vi "Teleop.vi"(10 "Match Info":T1={"Autonomous Elapsed Seconds"=0.0, "TeleOp Elapsed Seconds"=0.0, "Disabled Elapsed Seconds"=0.0, "Visited Autonomous"=FALSE, "Visited TeleOp"=FALSE, "Visited Disabled"=FALSE, "Autonomous Settings"={"Autonomous Style"=enum."Independent", "VI Refnum"=refnum}}, 11 "Call Context":T2) -> ()   [LabVIEW 2017]
doc: "This VI is called for each TeleOp packet received from the DS where the robot is not disabled. It is often used to read from the joysticks and update I/O or to update setpoints for timed control loops. It should complete and return within 20 milliseconds or it may miss DS packets."
uses:
  <vilib>/Rock Robotics/WPI/DriverStation/WPI_DriverStationDerivedRobotMode.ctl
  <vilib>/Rock Robotics/WPI/DriverStation/WPI_DriverStationMatch Info.ctl
  <vilib>/Rock Robotics/WPI/Utilities/WPI_GetSetVariantRefNum.vi
  <vilib>/Rock Robotics/Network Tables/NT Write Boolean Array.vi
  <vilib>/Rock Robotics/Network Tables/NT Write Numeric Array.vi
  <vilib>/Rock Robotics/Network Tables/NT Read Boolean.vi
  <vilib>/Rock Robotics/Network Tables/NT Read Number.vi
  Robot Global Data.vi
panel:
  out "Sample Slider 0":dbl(slide) scale=0.0..5.0
  out "Sample Boolean 1":bool
  out "Sample Boolean 0":bool
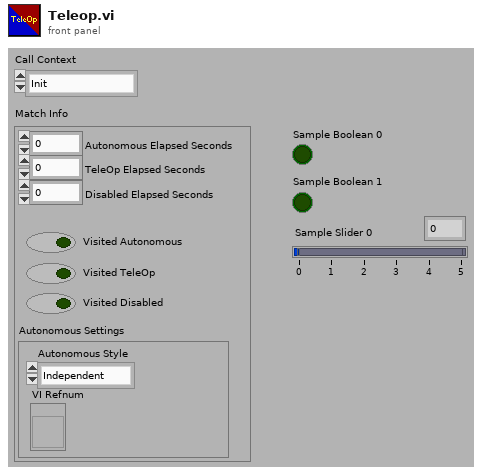
[diagram p1: front panel]
types:
  T1 = typedef "WPI_DriverStationMatch Info.ctl" = cluster{"Autonomous Elapsed Seconds":dbl, "TeleOp Elapsed Seconds":dbl, "Disabled Elapsed Seconds":dbl, "Visited Autonomous":bool, "Visited TeleOp":bool, "Visited Disabled":bool, "Autonomous Settings":cluster{"Autonomous Style":enum16{"Iterative", "Independent"}, "VI Refnum":refnum<vi>}}
  T2 = typedef "WPI_DriverStationDerivedRobotMode.ctl" = enum16{"Init", "Execute", "Stop"}
  T3 = typedef "WPI_MotorControlDeviceRef.ctl" = cluster{"DeviceStatus":errorcluster, "Type":T4, "PWM":cluster{"PWM Channel":T5, "DeadBand":T6}, "CAN":cluster{"Device Number":u8, "SetOutput VI Ref":variant, "GetOutput VI Ref":variant, "Enable VI Ref":variant, "Disable VI Ref":variant, "Data":variant}, "Invert":bool, "DIO PWM":cluster{"PWM \"Enable\" Channel":T5, "DIOChannel":T7, "PWM Rate":dbl}}
  T4 = typedef "WPI_MotorControlType.ctl" = enum16{"PWM", "CAN", "DIO PWM"}
  T5 = typedef "FPGA_DIOPWMChannel.ctl" = enum8{"PWM 0", "PWM 1", "PWM 2", "PWM 3", "PWM 4", "PWM 5", "PWM 6", "PWM 7", "PWM 8", "PWM 9", "PWM MXP 0", "PWM MXP 1", "PWM MXP 2", "PWM MXP 3", "PWM MXP 4", "PWM MXP 5", "PWM MXP 6", "PWM MXP 7", "PWM MXP 8", "PWM MXP 9", "Invalid"}
  T6 = typedef "WPI_PWMDeadband.ctl" = cluster{"Name":string, "maxPositivePwm":i32, "minPositivePwm":i32, "centerPwm":i32, "maxNegativePwm":i32, "minNegativePwm":i32, "angularRange":u16}
  T7 = typedef "FPGA_DIOChannel.ctl" = enum8{"DIO 0", "DIO 1", "DIO 2", "DIO 3", "DIO 4", "DIO 5", "DIO 6", "DIO 7", "DIO 8", "DIO 9", "DIO MXP 0", "DIO MXP 1", "DIO MXP 2", "DIO MXP 3", "DIO MXP 4", "DIO MXP 5", "DIO MXP 6", "DIO MXP 7", "DIO MXP 8", "DIO MXP 9", "DIO MXP 10", "DIO MXP 11", "DIO MXP 12", "DIO MXP 13", "DIO MXP 14", "DIO MXP 15", "SPI Port CS1", "SPI Port CS2", "SPI Port CS3", "SPI Port MISO", "SPI Port MOSI", "Invalid"}
  T8 = typedef "WPI_RobotDriveDevRef.ctl" = cluster{"DevStatus":errorcluster, "Motors[]":T3[], "Square Inputs":bool, "Max Output":dbl}
  T9 = typedef "WPI_JoystickDevRef.ctl" = cluster{"Device":T10}
  T10 = typedef "WPI_JoystickDeviceEnum.ctl" = enum16{"USB 0", "USB 1", "USB 2", "USB 3", "USB 4", "USB 5"}
  T11 = typedef "WPI_CompressorDevRef.ctl" = cluster{"DevStatus":errorcluster, "Pneumatics Control Module":u8}
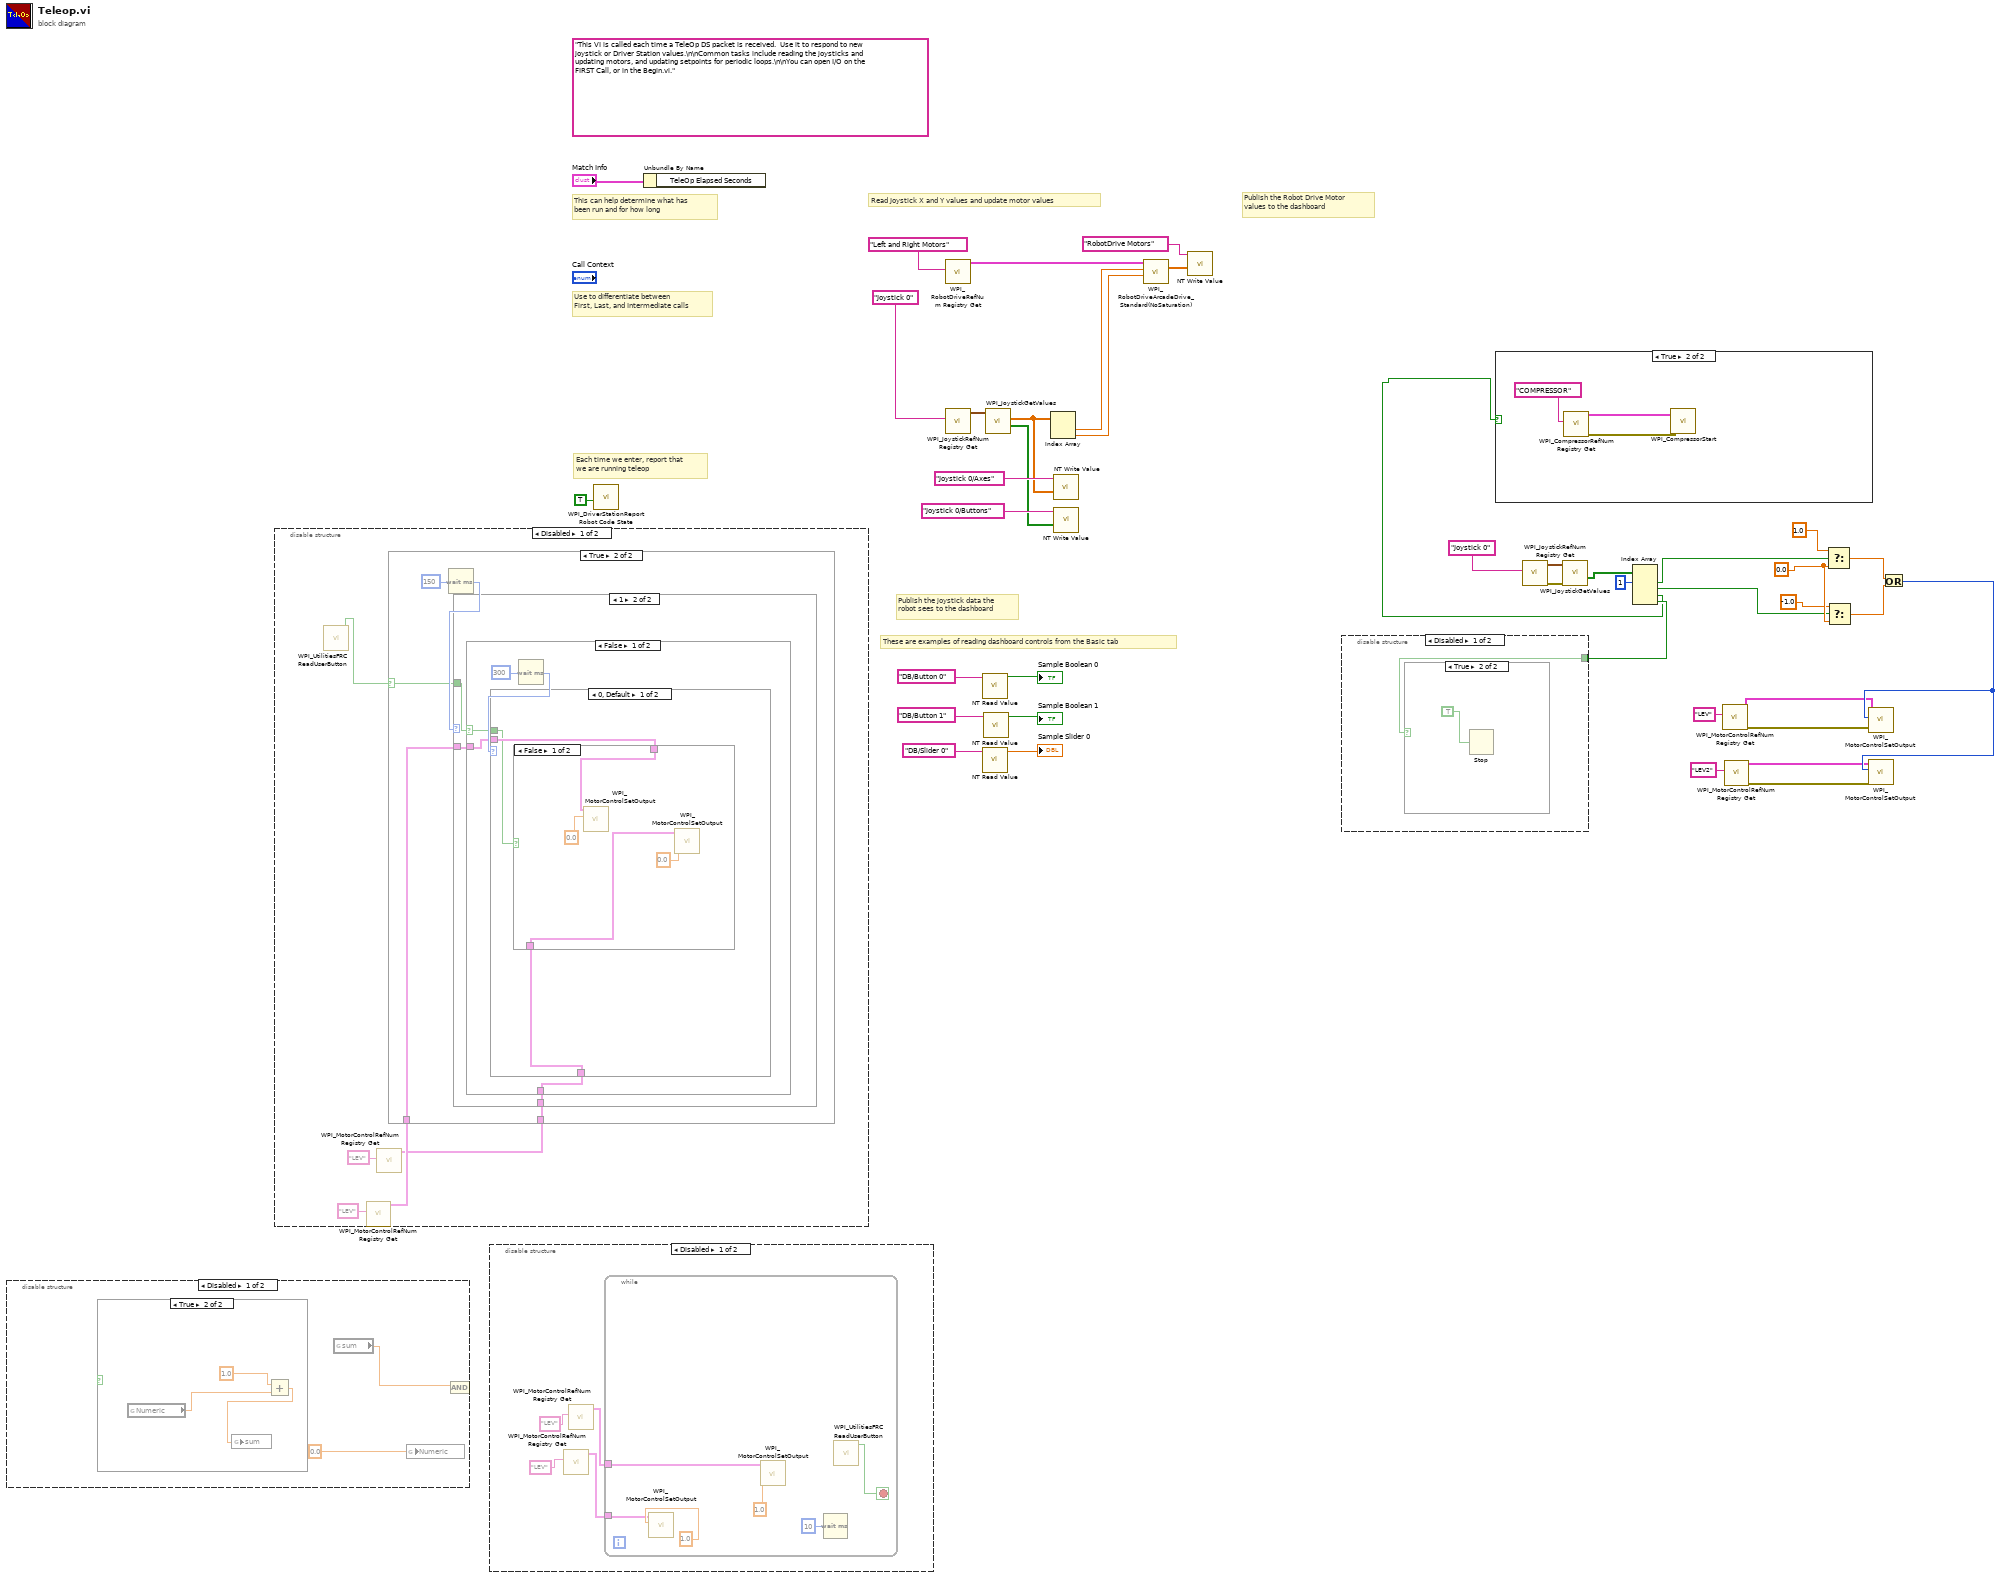
[diagram p0: block diagram]
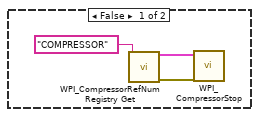
[diagram p4: hidden frame]
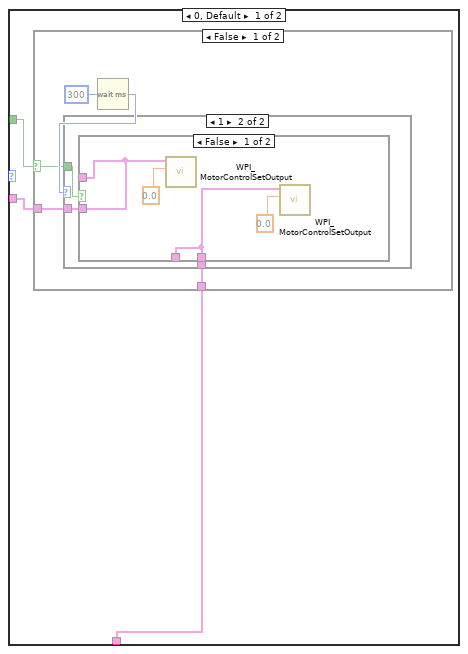
[diagram p9: hidden frame]
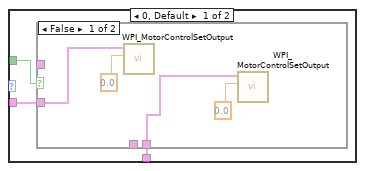
[diagram p10: hidden frame]
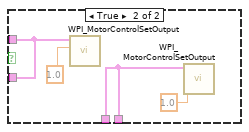
[diagram p11: hidden frame]
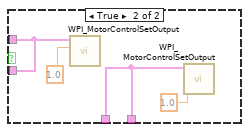
[diagram p12: hidden frame]
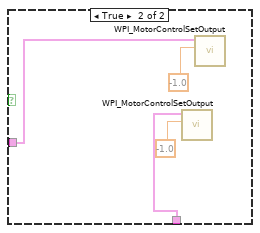
[diagram p13: hidden frame]
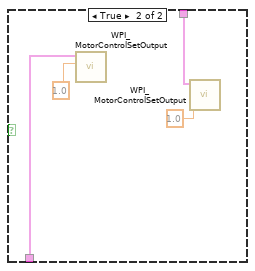
[diagram p14: hidden frame]
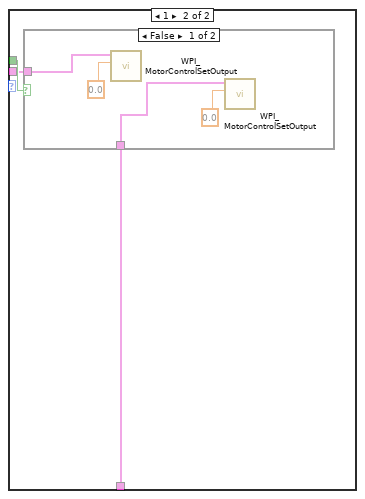
[diagram p15: hidden frame]
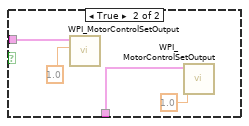
[diagram p16: hidden frame]
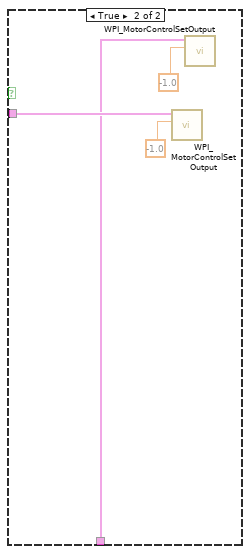
[diagram p17: hidden frame]
diagram:
  w16 = 0.0 ("t")
  (unwired) "This VI is called each time a TeleOp DS packet is received.  Use it to respond to new joystick or Driver Station values.\n\nCommon tasks include reading the joysticks and updating motors, and updating setpoints for periodic loops.\n\nYou can open I/O on the FIRST Call, or in the Begin.vi."
  # "Publish the Robot Drive Motor\nvalues to the dashboard"
  # "These are examples of reading dashboard controls from the Basic tab"
  # "Publish the joystick data the\nrobot sees to the dashboard"
  # "Each time we enter, report that\nwe are running teleop"
  # "Use to differentiate between\nFirst, Last, and Intermediate calls"
  # "This can help determine what has\nbeen run and for how long"
  # "Read Joystick X and Y values and update motor values"
  n1 = disable-structure shown="Disabled" {
    frame Disabled {
      n2 = case shown="True" {
        selector: _ -> [_ _]
        frame False {
        }
        frame True {
          n3 = global read "Robot Global Data.vi" "Numeric"() -> (w46:dbl)
          n4 = Add(x=1.0 ("Numeric"), y=w46) -> (x+y=w44:dbl)
          n5 = global write "Robot Global Data.vi" "sum"(w44) -> ()
        }
      }
      n6 = global read "Robot Global Data.vi" "sum"() -> (w42:dbl)
      n7 = global write "Robot Global Data.vi" "Numeric"(0.0 ("Numeric")) -> ()
      n8 = And(x=w42) -> ()  [unwired: 1 in, 1 out]
    }
    frame Enabled {
    }
  }
  n9 = disable-structure shown="Disabled" {
    frame Disabled {
      n10 = call <vilib>:"WPI_UtilitiesFRC ReadUserButton.vi"() -> ("User Button"=w51:bool)  [unwired: 10 in, 1 out]
      n11 = call <vilib>:"WPI_MotorControlRefNum Registry Get.vi"("refnum name"="LEV") -> ("MotorControlDevRef"=w48:T3)  [unwired: 9 in, 1 out]
      n12 = call <vilib>:"WPI_MotorControlRefNum Registry Get.vi"("refnum name"="LEV") -> ("MotorControlDevRef"=w47:T3)  [unwired: 9 in, 1 out]
      n13 = case shown="True" w51 {
        selector: w51 -> [_ w54]
        tunnel: w48 -> [_ w53]
        tunnel: w47 -> [_ w52]
        frame False {
        }
        frame True {
          n14 = Wait (ms)(milliseconds to wait=u32 150) -> (millisecond timer value=w56:u32)
          n15 = case shown="1" w56 {
            tunnel: w54 -> [w57 w93]
            tunnel: w53 -> [w59 w92]
            tunnel: w52 -> [w58 w91]
            frame 0, Default {
              n16 = case shown="False" w57 {
                selector: w57 -> [w62 _]
                tunnel: w59 -> [w61 w88]
                tunnel: w58 -> [w60 w87]
                frame False {
                  n17 = Wait (ms)(milliseconds to wait=u32 300) -> (millisecond timer value=w63:u32)
                  n18 = case shown="1" w63 {
                    tunnel: w62 -> [w67 w78]
                    tunnel: w61 -> [w66 w77]
                    tunnel: w60 -> [w65 w76]
                    frame 0, Default {
                      n19 = case shown="False" w67 {
                        tunnel: [_ w73] -> _
                        tunnel: [_ w72] -> _
                        tunnel: w66 -> [w69 w73]
                        tunnel: w65 -> [w68 w72]
                        frame False {
                          n20 = call <vilib>:"WPI_MotorControlSetOutput.vi"("Output"=0.0, "MotorControlDevRef"=w69) -> ()  [unwired: 7 in, 3 out]
                          n21 = call <vilib>:"WPI_MotorControlSetOutput.vi"("Output"=0.0, "MotorControlDevRef"=w68) -> ()  [unwired: 7 in, 3 out]
                        }
                        frame True {
                          n22 = call <vilib>:"WPI_MotorControlSetOutput.vi"("Output"=1.0, "MotorControlDevRef"=w73) -> ()  [unwired: 7 in, 3 out]
                          n23 = call <vilib>:"WPI_MotorControlSetOutput.vi"("Output"=1.0, "MotorControlDevRef"=w72) -> ()  [unwired: 7 in, 3 out]
                        }
                      }
                    }
                    frame 1 {
                      n24 = case shown="False" w78 {
                        tunnel: [w80 w83] -> _
                        tunnel: [w79 w84] -> _
                        tunnel: w77 -> [w80 w83]
                        tunnel: w76 -> [w79 w84]
                        frame False {
                          n25 = call <vilib>:"WPI_MotorControlSetOutput.vi"("Output"=0.0, "MotorControlDevRef"=w80) -> ()  [unwired: 7 in, 3 out]
                          n26 = call <vilib>:"WPI_MotorControlSetOutput.vi"("Output"=0.0, "MotorControlDevRef"=w79) -> ()  [unwired: 7 in, 3 out]
                        }
                        frame True {
                          n27 = call <vilib>:"WPI_MotorControlSetOutput.vi"("Output"=1.0, "MotorControlDevRef"=w83) -> ()  [unwired: 7 in, 3 out]
                          n28 = call <vilib>:"WPI_MotorControlSetOutput.vi"("Output"=1.0, "MotorControlDevRef"=w84) -> ()  [unwired: 7 in, 3 out]
                        }
                      }
                    }
                  }
                }
                frame True {
                  n29 = call <vilib>:"WPI_MotorControlSetOutput.vi"("Output"=-1.0, "MotorControlDevRef"=w87) -> ()  [unwired: 7 in, 3 out]
                  n30 = call <vilib>:"WPI_MotorControlSetOutput.vi"("Output"=-1.0, "MotorControlDevRef"=w88) -> ()  [unwired: 7 in, 3 out]
                }
              }
            }
            frame 1 {
              n31 = case shown="False" w93 {
                selector: w93 -> [w96 _]
                tunnel: w92 -> [w95 w123]
                tunnel: w91 -> [w94 w121]
                frame False {
                  n32 = Wait (ms)(milliseconds to wait=u32 300) -> (millisecond timer value=w97:u32)
                  n33 = case shown="0, Default" w97 {
                    tunnel: w96 -> [w99 w112]
                    tunnel: w95 -> [w100 w111]
                    tunnel: w94 -> [w101 w110]
                    frame 0, Default {
                      n34 = case shown="False" w99 {
                        tunnel: w101 -> [w103 w107]
                        tunnel: w100 -> [w102 w106]
                        frame False {
                          n35 = call <vilib>:"WPI_MotorControlSetOutput.vi"("Output"=0.0, "MotorControlDevRef"=w102) -> ()  [unwired: 7 in, 3 out]
                          n36 = call <vilib>:"WPI_MotorControlSetOutput.vi"("Output"=0.0, "MotorControlDevRef"=w103) -> ()  [unwired: 7 in, 3 out]
                        }
                        frame True {
                          n37 = call <vilib>:"WPI_MotorControlSetOutput.vi"("Output"=1.0, "MotorControlDevRef"=w107) -> ()  [unwired: 7 in, 3 out]
                          n38 = call <vilib>:"WPI_MotorControlSetOutput.vi"("Output"=1.0, "MotorControlDevRef"=w106) -> ()  [unwired: 7 in, 3 out]
                        }
                      }
                    }
                    frame 1 {
                      n39 = case shown="False" w112 {
                        tunnel: w111 -> [w113 w118]
                        tunnel: w110 -> [w114 w117]
                        frame False {
                          n40 = call <vilib>:"WPI_MotorControlSetOutput.vi"("Output"=0.0, "MotorControlDevRef"=w113) -> ()  [unwired: 7 in, 3 out]
                          n41 = call <vilib>:"WPI_MotorControlSetOutput.vi"("Output"=0.0, "MotorControlDevRef"=w114) -> ()  [unwired: 7 in, 3 out]
                        }
                        frame True {
                          n42 = call <vilib>:"WPI_MotorControlSetOutput.vi"("Output"=1.0, "MotorControlDevRef"=w118) -> ()  [unwired: 7 in, 3 out]
                          n43 = call <vilib>:"WPI_MotorControlSetOutput.vi"("Output"=1.0, "MotorControlDevRef"=w117) -> ()  [unwired: 7 in, 3 out]
                        }
                      }
                    }
                  }
                }
                frame True {
                  n44 = call <vilib>:"WPI_MotorControlSetOutput.vi"("Output"=-1.0, "MotorControlDevRef"=w123) -> ()  [unwired: 7 in, 3 out]
                  n45 = call <vilib>:"WPI_MotorControlSetOutput.vi"("Output"=-1.0, "MotorControlDevRef"=w121) -> ()  [unwired: 7 in, 3 out]
                }
              }
            }
          }
        }
      }
    }
    frame Enabled {
    }
  }
  n46 = disable-structure shown="Disabled" {
    frame Disabled {
      n47 = call <vilib>:"WPI_MotorControlRefNum Registry Get.vi"("refnum name"="LEV") -> ("MotorControlDevRef"=w125:T3)  [unwired: 9 in, 1 out]
      n48 = call <vilib>:"WPI_MotorControlRefNum Registry Get.vi"("refnum name"="LEV") -> ("MotorControlDevRef"=w126:T3)  [unwired: 9 in, 1 out]
      n49 = while {
        tunnel: w126 -> [w131]
        tunnel: w125 -> [w130]
        stop <- w134 stop-if-true
        n50 = call <vilib>:"WPI_MotorControlSetOutput.vi"("Output"=1.0, "MotorControlDevRef"=w130) -> ()  [unwired: 7 in, 3 out]
        n51 = call <vilib>:"WPI_MotorControlSetOutput.vi"("Output"=1.0, "MotorControlDevRef"=w131) -> ()  [unwired: 7 in, 3 out]
        n52 = Wait (ms)(milliseconds to wait=u32 10) -> ()  [unwired: 1 out]
        n53 = call <vilib>:"WPI_UtilitiesFRC ReadUserButton.vi"() -> ("User Button"=w134:bool)  [unwired: 10 in, 1 out]
      }
    }
    frame Enabled {
    }
  }
  n54 = call <vilib>:"WPI_DriverStationReport Robot Code State.vi"("TeleOp"=TRUE ("Autonomous")) -> ()  [unwired: 10 in, 1 out]
  n55 = Unbundle By Name("Match Info") -> ()  [unwired: 1 out]
  n56 = call <vilib>:"WPI_RobotDriveRefNum Registry Get.vi"("refnum name"="Left and Right Motors") -> ("RobotDriveDevRef"=w39:T8)  [unwired: 1 in, 9 out]
  n57 = call <vilib>:"WPI_JoystickRefNum Registry Get.vi"("refnum name"="Joystick 0") -> ("JoystickDevRef"=w36:T9)  [unwired: 1 in, 9 out]
  n58 = call-poly <vilib>:"NT Read Value.vi"("Name"="DB/Button 0" ("refnum name")) -> ("Boolean"=→"Sample Boolean 0":bool)  [unwired: 9 in, 1 out]
  n59 = call-poly <vilib>:"NT Read Value.vi"("Name"="DB/Slider 0" ("refnum name")) -> ("Numeric"=→"Sample Slider 0":dbl)  [unwired: 9 in, 1 out]
  n60 = call-poly <vilib>:"NT Read Value.vi"("Name"="DB/Button 1" ("refnum name")) -> ("Boolean"=→"Sample Boolean 1":bool)  [unwired: 9 in, 1 out]
  n61 = call <vilib>:"WPI_JoystickGetValues.vi"("JoystickDevRef"=w36) -> ("Buttons"=w3:bool[], "Axes"=w31:dbl[])  [unwired: 6 in, 3 out]
  n62 = Index Array(array=w31) -> (element #1=w38:dbl, element #2=w34:dbl)  [unwired: 2 in]
  n63 = call-poly <vilib>:"NT Write Value.vi"("Numeric Array"=w31, "Name"="Joystick 0/Axes") -> ()  [unwired: 9 in, 1 out]
  n64 = call-poly <vilib>:"NT Write Value.vi"("Boolean Array"=w3, "Name"="Joystick 0/Buttons") -> ()  [unwired: 9 in, 1 out]
  n65 = call <vilib>:"WPI_RobotDriveArcadeDrive_Standard(NoSaturation).vi"("Y axis value"=w34, "X axis value"=w38, "RobotDriveDevRef"=w39) -> ("Motor Values"=w24:dbl[])  [unwired: 1 in, 7 out]
  n66 = call-poly <vilib>:"NT Write Value.vi"("Numeric Array"=w24, "Name"="RobotDrive Motors") -> ()  [unwired: 9 in, 1 out]
  n67 = call <vilib>:"WPI_JoystickRefNum Registry Get.vi"("refnum name"="Joystick 0") -> ("error out"=w19:errorcluster, "JoystickDevRef"=w22:T9)  [unwired: 1 in, 8 out]
  n68 = call <vilib>:"WPI_JoystickGetValues.vi"("error in (no error)"=w19, "JoystickDevRef"=w22) -> ("Buttons"=w20:bool[])  [unwired: 5 in, 4 out]
  n69 = Index Array(array=w20, index #1=1 ("index")) -> (element #1=w5:bool, element #2=w4:bool, element #3=w1:bool, element #4=w2:bool)  [unwired: 3 in]
  n70 = disable-structure shown="Disabled" {
    disable-tunnel: w2 -> [w135 _]
    frame Disabled {
      n71 = case shown="True" w135 {
        frame False {
        }
        frame True {
          n72 = Stop(stop? (T)=TRUE) -> ()
        }
      }
    }
    frame Enabled {
    }
  }
  n73 = case shown="True" w1 {
    frame False {
      n74 = call <vilib>:"WPI_CompressorRefNum Registry Get.vi"("refnum name"="COMPRESSOR") -> ("error out"=w139:errorcluster, "CompressorDevRef"=w138:T11)  [unwired: 9 in]
      n75 = call <vilib>:"WPI_CompressorStop.vi"("error in (no error)"=w139, "CompressorDevRef"=w138) -> ()  [unwired: 8 in, 2 out]
    }
    frame True {
      n76 = call <vilib>:"WPI_CompressorRefNum Registry Get.vi"("refnum name"="COMPRESSOR") -> ("error out"=w140:errorcluster, "CompressorDevRef"=w141:T11)  [unwired: 9 in]
      n77 = call <vilib>:"WPI_CompressorStart.vi"("error in (no error)"=w140, "CompressorDevRef"=w141) -> ()  [unwired: 8 in, 2 out]
    }
  }
  n78 = call <vilib>:"WPI_MotorControlRefNum Registry Get.vi"("refnum name"="LEV") -> ("error out"=w9:errorcluster, "MotorControlDevRef"=w8:T3)  [unwired: 9 in]
  n79 = call <vilib>:"WPI_MotorControlRefNum Registry Get.vi"("refnum name"="LEV2") -> ("error out"=w10:errorcluster, "MotorControlDevRef"=w11:T3)  [unwired: 9 in]
  n80 = Select(t=1.0, s=w5, f=w16) -> (s? t:f=w14:dbl)
  n81 = Select(t=-1.0, s=w4, f=w16) -> (s? t:f=w13:dbl)
  n82 = Or(x=w14, y=w13) -> (x .or. y?=w12:i32)
  n83 = call <vilib>:"WPI_MotorControlSetOutput.vi"("error in (no error)"=w9, "Output"=w12, "MotorControlDevRef"=w8) -> ()  [unwired: 6 in, 3 out]
  n84 = call <vilib>:"WPI_MotorControlSetOutput.vi"("error in (no error)"=w10, "Output"=w12, "MotorControlDevRef"=w11) -> ()  [unwired: 6 in, 3 out]
